vi "GridGenerator.vi"(1 "starty":i16, 2 "startx":i16, 3 "stepy":i16=1, 4 "samplesy":i32=128, 5 "stepx":i16=1, 6 "samplesx":i32=128) -> (0 "appended array":dbl[][](array[numeric]))   [LabVIEW 2015]
uses:
  <vilib>/Analysis/1siggen.llb/Ramp Pattern by Samples.vi
  <vilib>/Analysis/NI_AALBase.lvlib
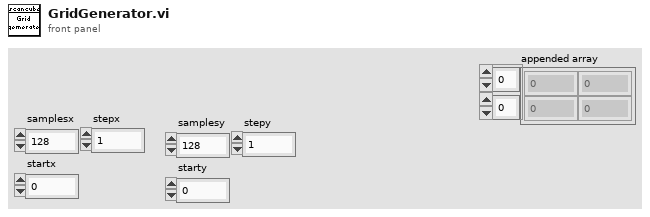
[diagram p1: front panel]
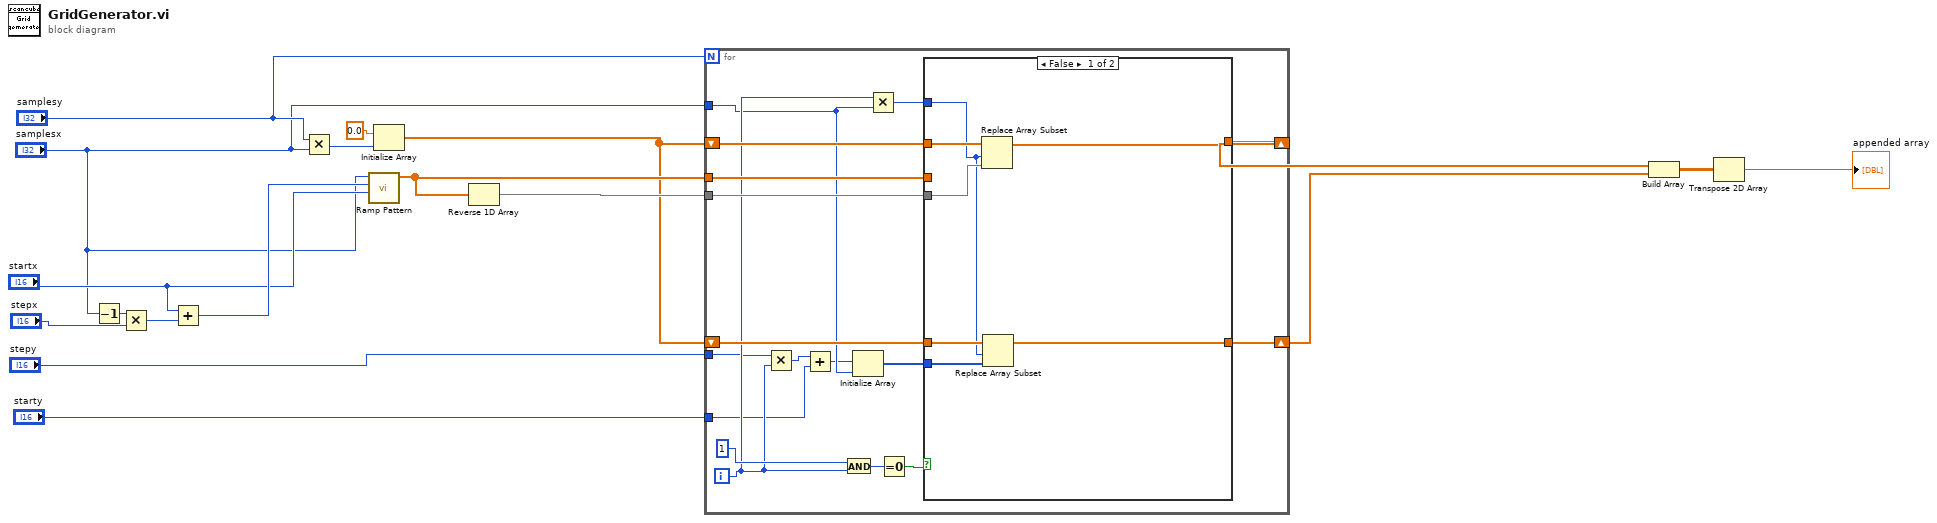
[diagram p0: block diagram]
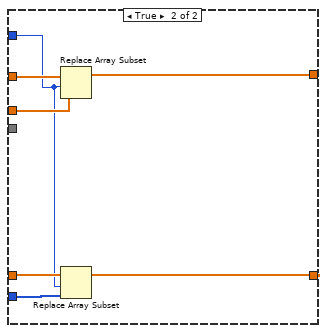
[diagram p2: hidden frame]
diagram:
  n1 = Decrement(x="samplesx") -> (x-1=w14:i32)
  n2 = Multiply(x=w14, y="stepx") -> (x*y=w17:i32)
  n3 = Add(x="startx", y=w17) -> (x+y=w16:i32)
  n4 = Multiply(x="samplesy", y="samplesx") -> (x*y=w4:i32)
  n5 = call-poly <vilib>:"Ramp Pattern.vi"("start"="startx", "end"=w16, "samples"="samplesx") -> ("Ramp Pattern"=w12:dbl[])  [unwired: 7 in, 1 out]
  n6 = Initialize Array(0.0 ("element"), w4) -> (w10:dbl[])
  n7 = Reverse 1D Array(array=w12) -> (reversed array=w11:dbl[])
  n8 = for {
    N: "samplesy" -> [_]
    shift-right: [w31] -> w8
    shift-left: w10 -> [w32]
    tunnel: "samplesx" -> [w24]
    tunnel: w12 -> [w30]
    tunnel: w11 -> [w29]
    shift-right: [w22] -> w7
    shift-left: w10 -> [w28]
    tunnel: "stepy" -> [w23]
    tunnel: "starty" -> [w19]
    i -> [w25]
    n9 = Multiply(x=w23, y=w25) -> (x*y=w21:i32)
    n10 = Add(x=w21, y=w19) -> (x+y=w20:i32)
    n11 = And(x=1, y=w25) -> (x .and. y?=w34:i32)
    n12 = Initialize Array(w20, w24) -> (w26:i32[])
    n13 = Multiply(x=w25, y=w24) -> (x*y=w27:i32)
    n14 = Equal To 0?(x=w34) -> (x = 0?=w33:bool)
    n15 = case shown="False" w33 {
      tunnel: w32 -> [w42 w49]
      tunnel: [w41 w48] -> w31
      tunnel: w27 -> [w37 w44]
      tunnel: w30 -> [_ w47]
      tunnel: w29 -> [w40 _]
      tunnel: w28 -> [w39 w46]
      tunnel: w26 -> [w36 w45]
      tunnel: [w38 w43] -> w22
      frame False {
        n16 = Replace Array Subset(array=w42, new element=w40, index=w37) -> (w41:dbl[])
        n17 = Replace Array Subset(array=w39, new element=w36, index=w37) -> (w38:dbl[])
      }
      frame True {
        n18 = Replace Array Subset(array=w49, new element=w47, index=w44) -> (w48:dbl[])
        n19 = Replace Array Subset(array=w46, new element=w45, index=w44) -> (w43:dbl[])
      }
    }
  }
  n20 = Build Array(w8, w7) -> (w2:dbl[][])
  n21 = Transpose 2D Array(2D array=w2) -> (transposed array=→"appended array":dbl[][])
